vi "tdscheck.vi"(0 "VISA Port In":refnum<visa-resource-name>, 1 "Error In (No Error)":errorcluster) -> (2 "VISA Port Out":refnum<visa-resource-name>, 3 "busy":bool, 4 "Error Out":errorcluster)   [LabVIEW 2011]
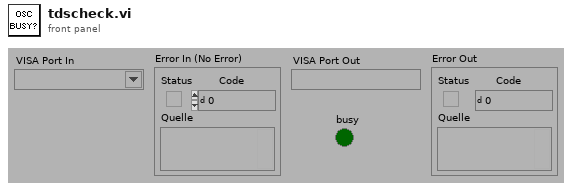
[diagram p1: front panel]
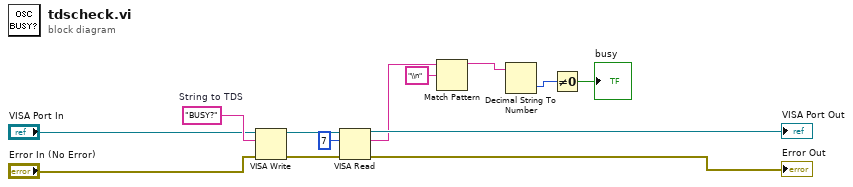
[diagram p0: block diagram]
diagram:
  w13 = "BUSY?"  # String to TDS
  n1 = VISA Write(VISA resource name="VISA Port In", write buffer=w13, error in (no error)="Error In (No Error)") -> (VISA resource name out=w10:refnum<visa-resource-name>, error out=w9:errorcluster)  [unwired: 1 out]
  n2 = VISA Read(VISA resource name=w10, byte count=u32 7, error in (no error)=w9) -> (VISA resource name out=→"VISA Port Out":refnum<visa-resource-name>, read buffer=w5:string, error out=→"Error Out":errorcluster)  [unwired: 1 out]
  n3 = Match Pattern(string=w5, regular expression="\\n") -> (before substring=w1:string)  [unwired: 1 in, 3 out]
  n4 = Decimal String To Number(string=w1) -> (number=w3:i32)  [unwired: 2 in, 1 out]
  n5 = Not Equal To 0?(x=w3) -> (x != 0?=→"busy":bool)
